vi "ROI entry screen-Apply variable resolution_retd-07022020.vi"(5 "XY Coordinates":i32[](array[numeric]), 7 "Col":i32, 8 "error in (no error)":errorcluster, 9 "Frame Size (original)":dbl, 10 "FOV (original)":dbl, 11 "ROI Variable resolution info":T1) -> (0 "error out":errorcluster, 1 "No of lines in ROI":i32, 2 "X pixels":dbl, 3 "ROI Variable resolution info O/P":T1, 4 "Angle (deg)":dbl, 6 "Pixels in ROI":i32)   [LabVIEW 2020]
uses:
  Typedefs/ROI Variable resolution info.ctl
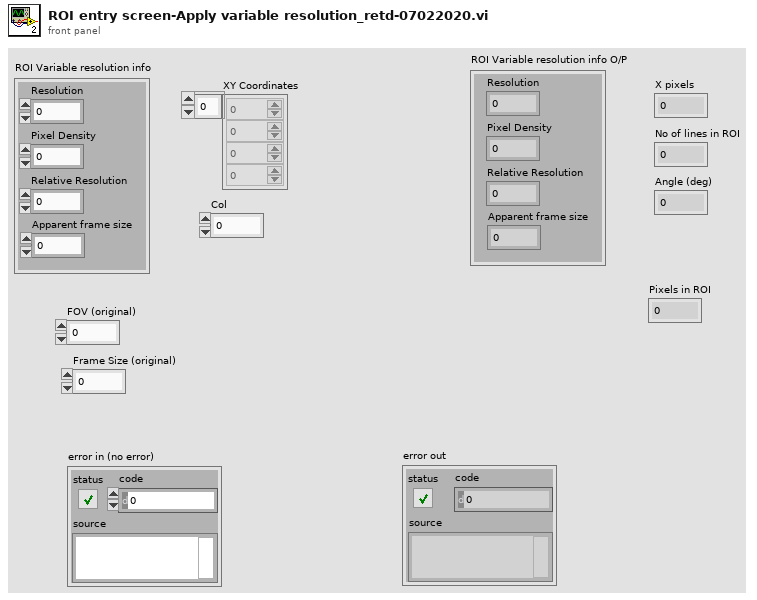
[diagram p1: front panel]
types:
  T1 = typedef "ROI Variable resolution info.ctl" = cluster{"Resolution":dbl, "Pixel Density":dbl, "Relative Resolution":dbl, "Apparent frame size":dbl}
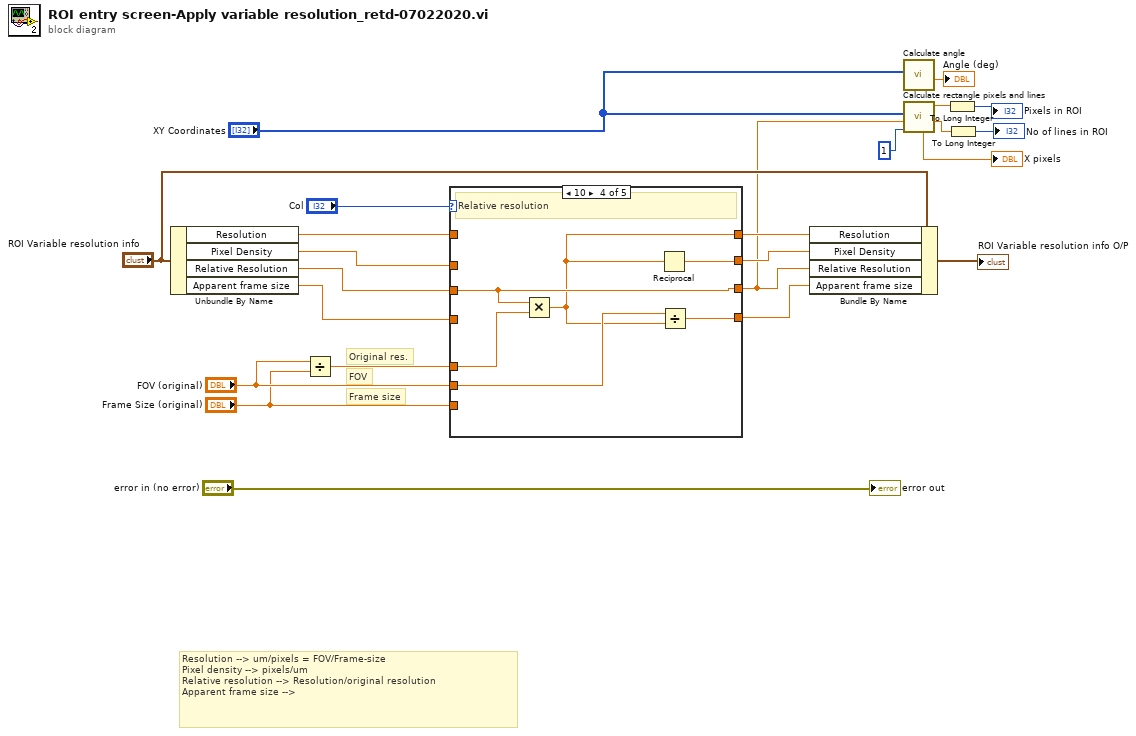
[diagram p0: block diagram]
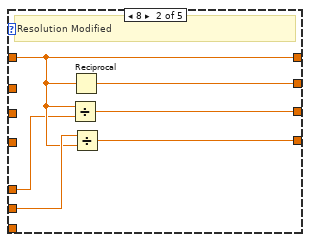
[diagram p3: hidden frame]
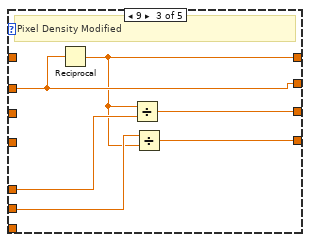
[diagram p4: hidden frame]
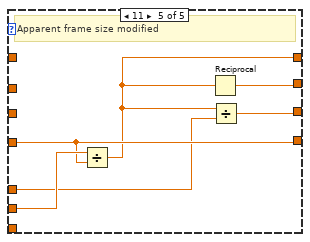
[diagram p5: hidden frame]
diagram:
  # "Frame size"
  # "FOV"
  # "Original res."
  # "Resolution --> um/pixels = FOV/Frame-size\nPixel density --> pixels/um\nRelative resolution --> Resolution/original resolution\nApparent frame size -->"
  n1 = Unbundle By Name("ROI Variable resolution info") -> ("Resolution"=w11:dbl, "Pixel Density"=w10:dbl, "Relative Resolution"=w9:dbl, "Apparent frame size"=w8:dbl)
  n2 = Divide(x="FOV (original)", y="Frame Size (original)") -> (x/y=w19:dbl)
  n3 = case shown="10" "Col" {
    tunnel: w11 -> [w27 w30 _ _ _]
    tunnel: [w26 w33 w37 w44 w49] -> w5
    tunnel: [w27 w30 w36 w41 w48] -> w6
    tunnel: w10 -> [w26 _ w37 _ _]
    tunnel: w9 -> [w25 _ _ w43 _]
    tunnel: "FOV (original)" -> [_ w32 w39 w42 w51]
    tunnel: [w24 w31 w34 w40 w50] -> w3
    tunnel: w19 -> [_ w29 w38 w45 w47]
    tunnel: [w25 w28 w35 w43 w46] -> w4
    tunnel: w8 -> [w24 _ _ _ w50]
    tunnel: "Frame Size (original)" -> [_ _ _ _ _]
    frame Default {
    }
    frame 8 {
      # "Resolution Modified"
      n4 = Divide(x=w30, y=w29) -> (x/y=w28:dbl)
      n5 = Reciprocal(x=w30) -> (1/x=w33:dbl)
      n6 = Divide(x=w32, y=w30) -> (x/y=w31:dbl)
    }
    frame 9 {
      # "Pixel Density Modified"
      n7 = Reciprocal(x=w37) -> (1/x=w36:dbl)
      n8 = Divide(x=w36, y=w38) -> (x/y=w35:dbl)
      n9 = Divide(x=w39, y=w36) -> (x/y=w34:dbl)
    }
    frame 10 {
      # "Relative resolution"
      n10 = Multiply(x=w43, y=w45) -> (x*y=w41:dbl)
      n11 = Reciprocal(x=w41) -> (1/x=w44:dbl)
      n12 = Divide(x=w42, y=w41) -> (x/y=w40:dbl)
    }
    frame 11 {
      # "Apparent frame size modified"
      n13 = Divide(x=w51, y=w50) -> (x/y=w48:dbl)
      n14 = Reciprocal(x=w48) -> (1/x=w49:dbl)
      n15 = Divide(x=w48, y=w47) -> (x/y=w46:dbl)
    }
  }
  n16 = Bundle By Name(cluster="ROI Variable resolution info", "Resolution"=w6, "Pixel Density"=w5, "Relative Resolution"=w4, "Apparent frame size"=w3) -> (→"ROI Variable resolution info O/P":T1)
  n17 = call "Calculate angle.vi"("XY Coordinates"="XY Coordinates") -> ("Angle (deg)"=→"Angle (deg)":dbl)  [unwired: 10 in]
  n18 = call "Calculate rectangle pixels and lines.vi"("No of Z planes"=1, "Resolution multiplier"=w4, "XY Coordinates (zero based)"="XY Coordinates") -> ("Number of lines (scaled)"=w15:dbl, "Pixels in ROI"=w16:dbl, "X pixels"=→"X pixels":dbl)  [unwired: 6 in]
  n19 = To Long Integer(number=w16) -> (32bit integer=→"Pixels in ROI":i32)
  n20 = To Long Integer(number=w15) -> (32bit integer=→"No of lines in ROI":i32)
  "error out" <- "error in (no error)"
